vi "string_to_mV_Rev_03.vi"(0 "Received HEX":string, 1 "Input Char":string, 2 "Nmbr_of_datasamples":dbl=128.0) -> (3 "minval":dbl, 4 "Waveform Graph":dbl[](graph), 5 "maxval":dbl, 6 "dataave":dbl, 7 "mV":dbl)   [LabVIEW 2012]
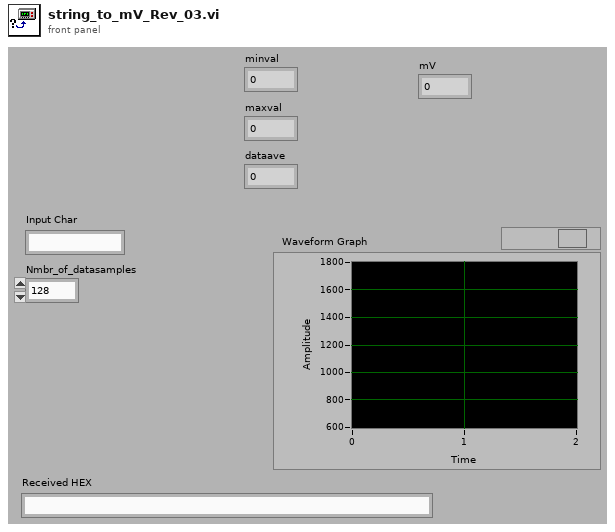
[diagram p1: front panel]
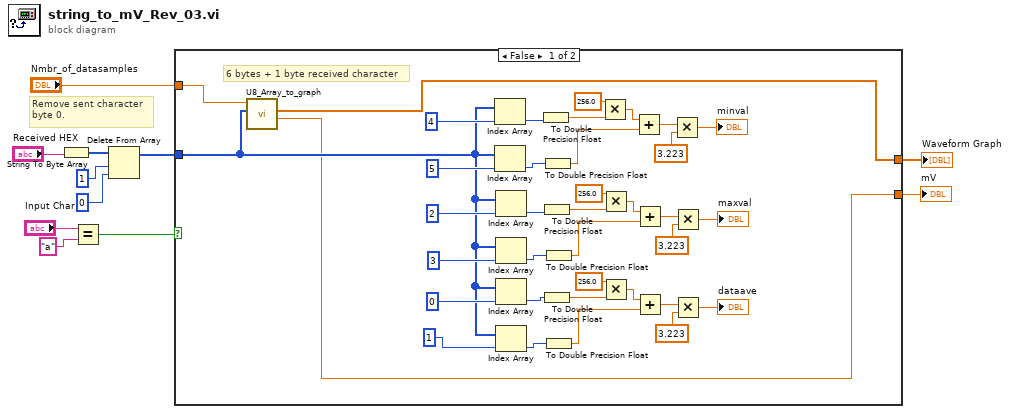
[diagram p0: block diagram]
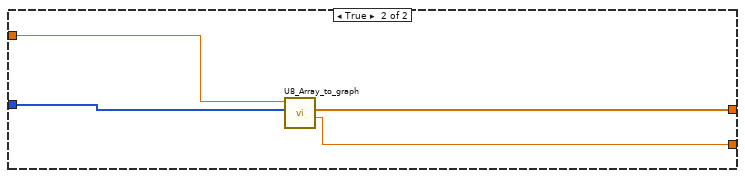
[diagram p2: hidden frame]
diagram:
  # "Remove sent character\nbyte 0."
  n1 = String To Byte Array(string="Received HEX") -> (unsigned byte array=w7:u8[])
  n2 = Equal?(x="Input Char", y="a") -> (x = y?=w4:bool)
  n3 = Delete From Array(array=w7, length=1, index=0) -> (array with subset deleted=w5:u8[])  [unwired: 1 out]
  n4 = case shown="False" w4 {
    tunnel: w5 -> [w14 w52]
    tunnel: "Nmbr_of_datasamples" -> [w15 w51]
    tunnel: [w13 w50] -> w2
    tunnel: [w12 w49] -> w1
    frame False {
      # "6 bytes + 1 byte received character"
      n5 = call "U8_Array_to_graph.vi"("Array In"=w14, "Nmbr_of_datasamples"=w15) -> ("mV"=w12:dbl, "Waveform Graph"=w13:dbl[])  [unwired: 7 in, 1 out]
      n6 = Index Array(array=w14, index=4) -> (element=w21:u8)
      n7 = Index Array(array=w14, index=5) -> (element=w18:u8)
      n8 = Index Array(array=w14, index=2) -> (element=w19:u8)
      n9 = Index Array(array=w14, index=3) -> (element=w20:u8)
      n10 = Index Array(array=w14, index=0) -> (element=w16:u8)
      n11 = Index Array(array=w14, index=1) -> (element=w17:u8)
      n12 = To Double Precision Float(number=w21) -> (double precision float=w30:dbl)
      n13 = To Double Precision Float(number=w19) -> (double precision float=w39:dbl)
      n14 = To Double Precision Float(number=w16) -> (double precision float=w47:dbl)
      n15 = To Double Precision Float(number=w18) -> (double precision float=w31:dbl)
      n16 = To Double Precision Float(number=w20) -> (double precision float=w40:dbl)
      n17 = To Double Precision Float(number=w17) -> (double precision float=w48:dbl)
      n18 = Multiply(x=256.0, y=w30) -> (x*y=w27:dbl)
      n19 = Multiply(x=256.0, y=w39) -> (x*y=w36:dbl)
      n20 = Multiply(x=256.0, y=w47) -> (x*y=w44:dbl)
      n21 = Add(x=w27, y=w31) -> (x+y=w28:dbl)
      n22 = Add(x=w36, y=w40) -> (x+y=w37:dbl)
      n23 = Add(x=w44, y=w48) -> (x+y=w45:dbl)
      n24 = Multiply(x=w28, y=3.223) -> (x*y=→"minval":dbl)
      n25 = Multiply(x=w37, y=3.223) -> (x*y=→"maxval":dbl)
      n26 = Multiply(x=w45, y=3.223) -> (x*y=→"dataave":dbl)
    }
    frame True {
      n27 = call "U8_Array_to_graph.vi"("Array In"=w52, "Nmbr_of_datasamples"=w51) -> ("mV"=w49:dbl, "Waveform Graph"=w50:dbl[])  [unwired: 7 in, 1 out]
    }
  }
  "mV" <- w1
  "Waveform Graph" <- w2
